vi "TAT_Com_PLC.vi"() -> ()   [LabVIEW 2017]
uses:
  Controls/PLC_Comm_State.ctl
  <vilib>/NI/Modbus Library/API/Master/Modbus Master.lvclass
  <vilib>/NI/Modbus Library/API/Wrapper/Create TCP Master.vi
  Global/PLC_to_Auto.vi
  <vilib>/NI/Modbus Library/API/Wrapper/API Main.lvlib
panel:
  out "PLC IP Address":string
  out "error out 2":errorcluster
  out "error IO":errorcluster
  in  "stop 2":bool
  out "PLC STATUS station 2":bool
  out "error IO 2":errorcluster
  out "Latch Error Case":errorcluster
  out "I/O SCREEN":bool[](array[boolean])
  out "error out":errorcluster
  in  "PLC STATUS station 1":bool
  in  "error in":errorcluster
  in  "stop":bool
  # "STATION 1"
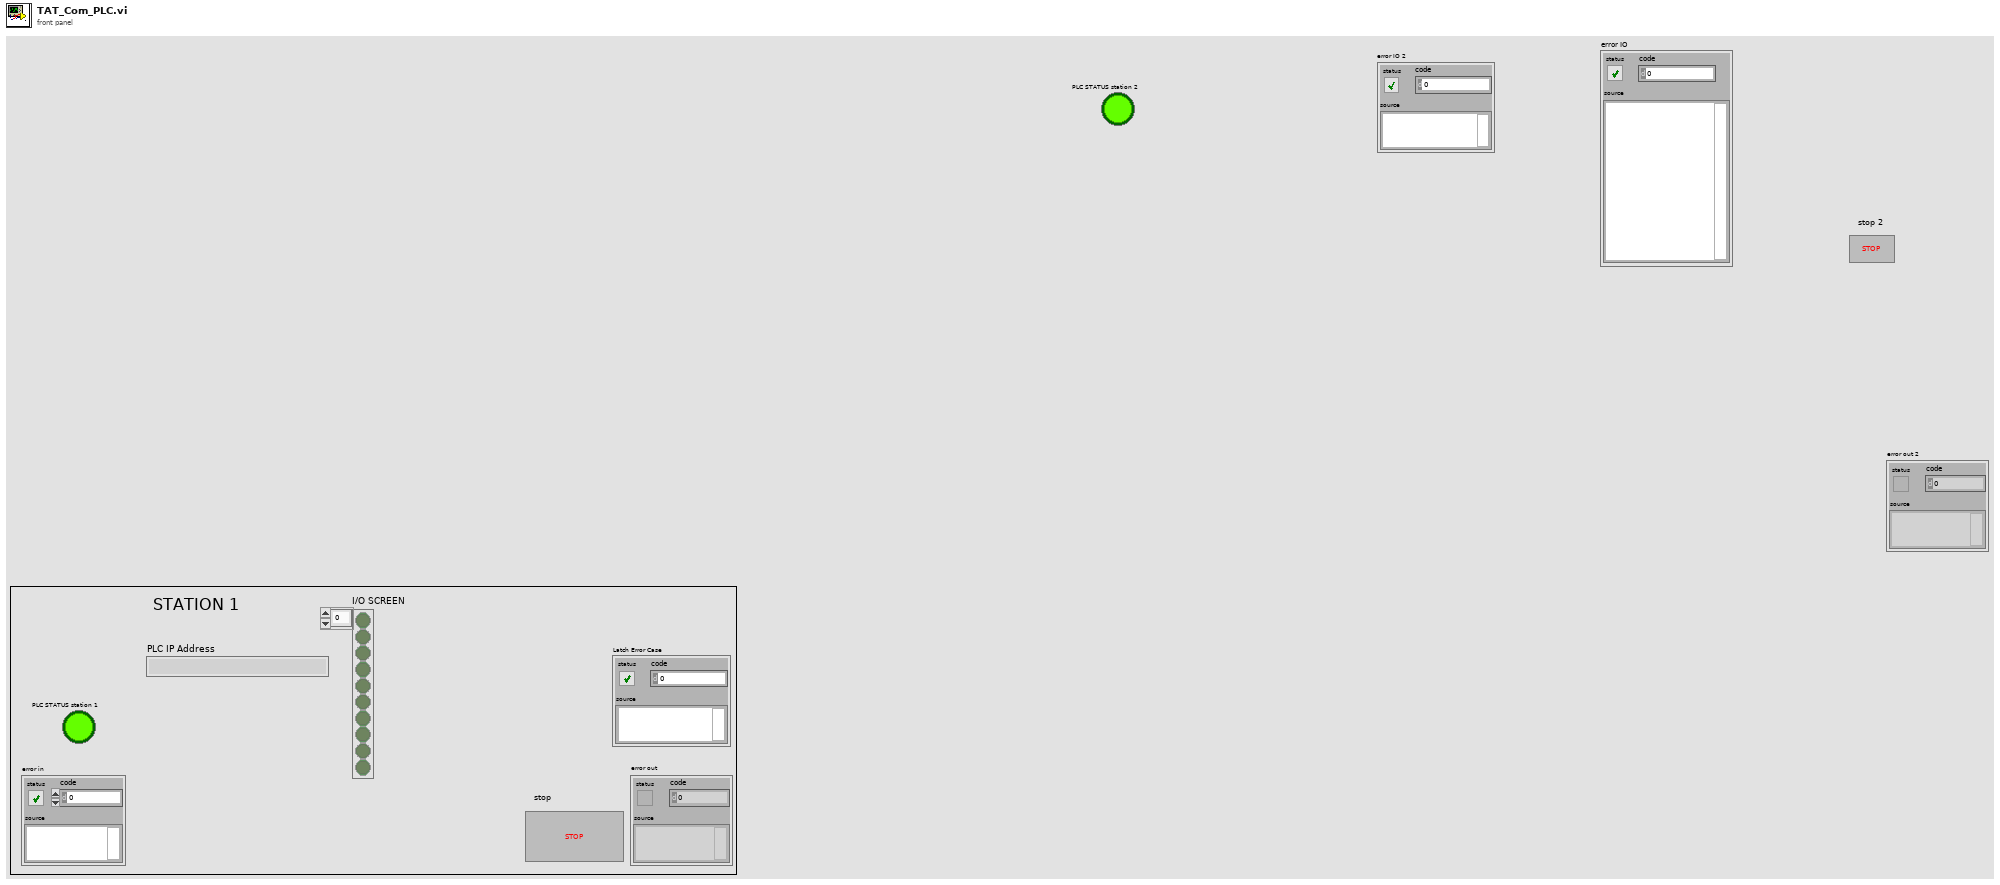
[diagram p1: front panel]
types:
  T1 = typedef "PLC_Comm_State.ctl" = enum16{"Int", "Connect", "Write", "Write2", "Write3", "Read", "Read2", "Read3", "Error", "Disconnect"}
  T2 = enum32{"invalid app kind", "Development System", "Run Time System", "Student Edition", "Embedded LabVIEW", "Evaluation", "Custom"}
  T3 = cluster{"Printer IP":string, "PLC IP Address":string, "Scanner Com":refnum<visa-resource-name>}
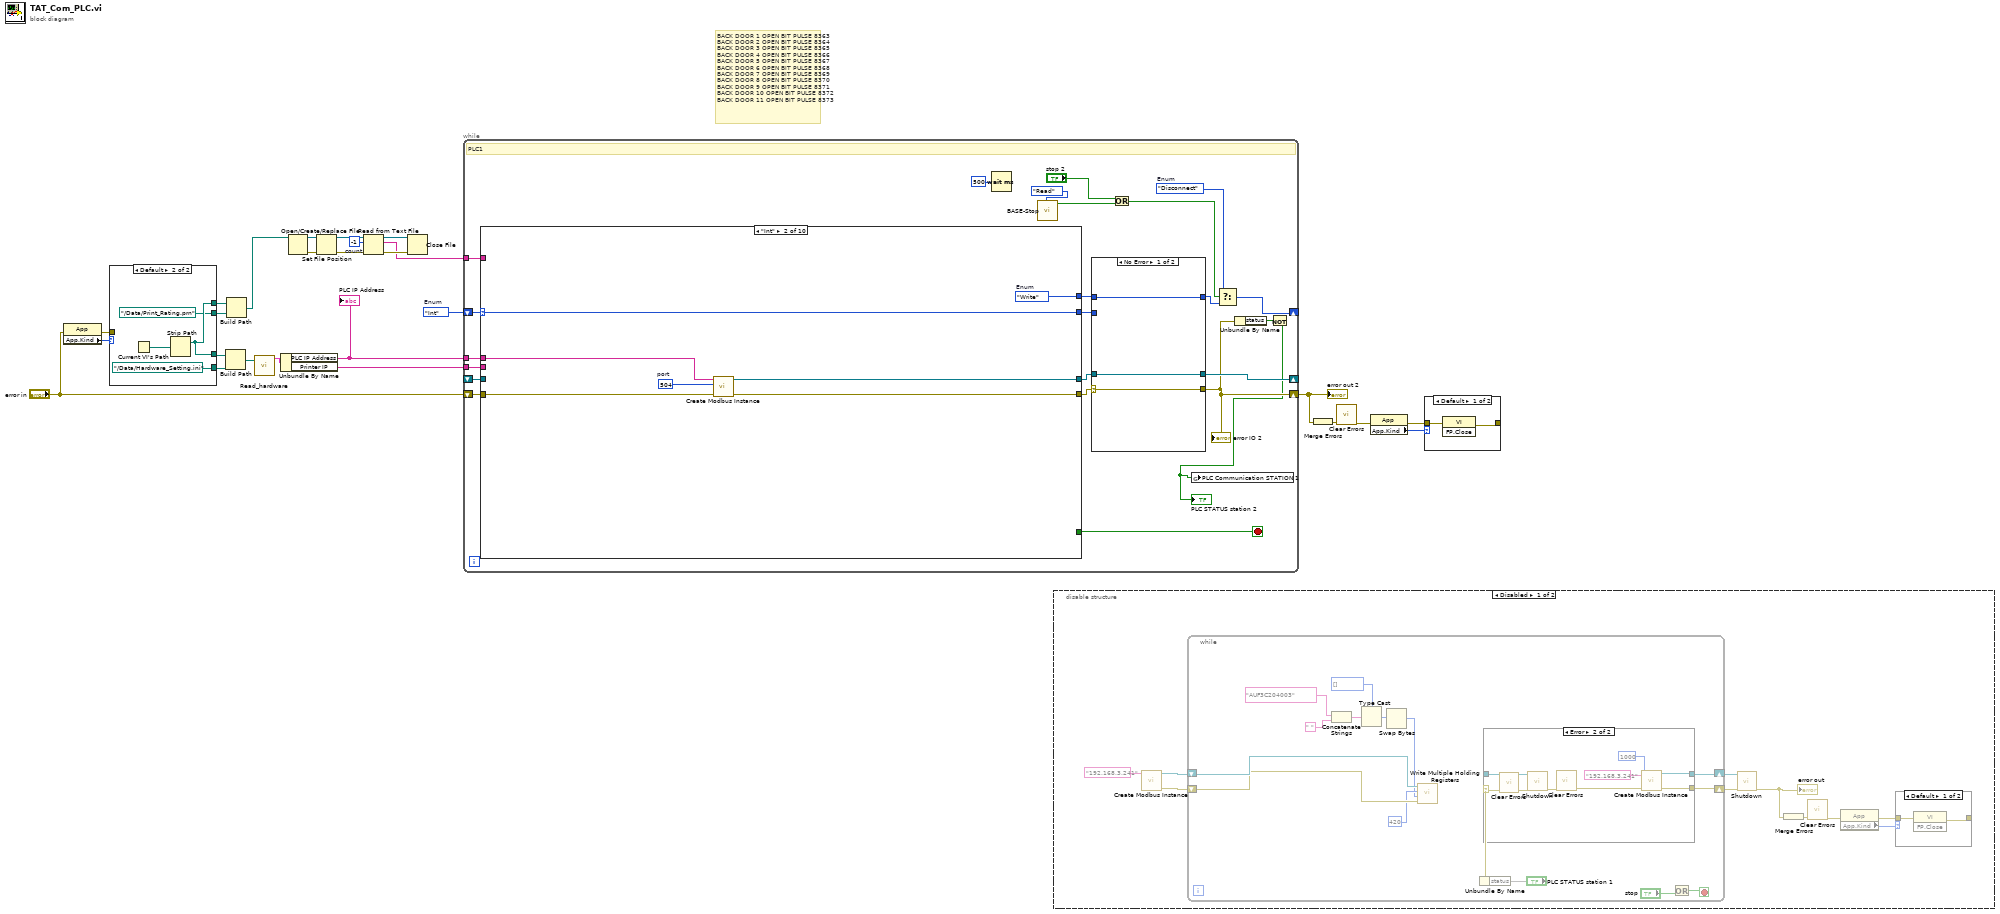
[diagram p0: block diagram]
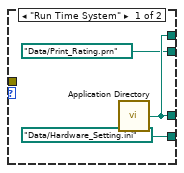
[diagram p2: hidden frame]
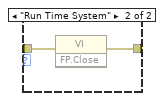
[diagram p4: hidden frame]
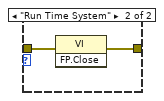
[diagram p6: hidden frame]
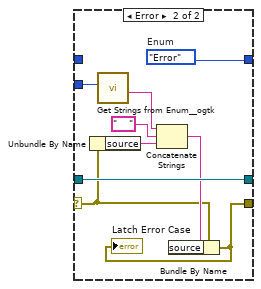
[diagram p7: hidden frame]
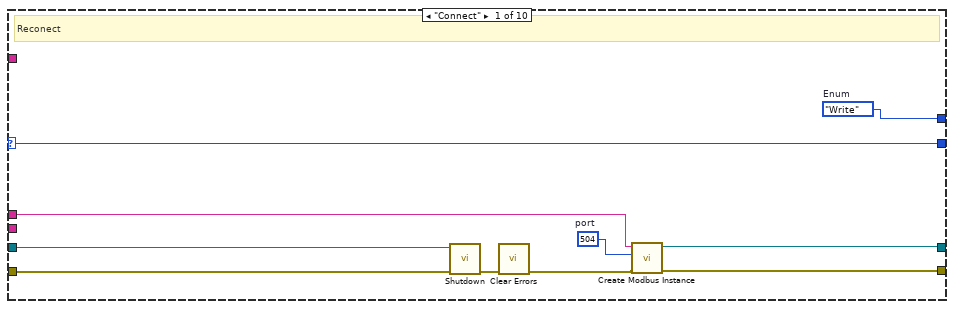
[diagram p8: hidden frame]
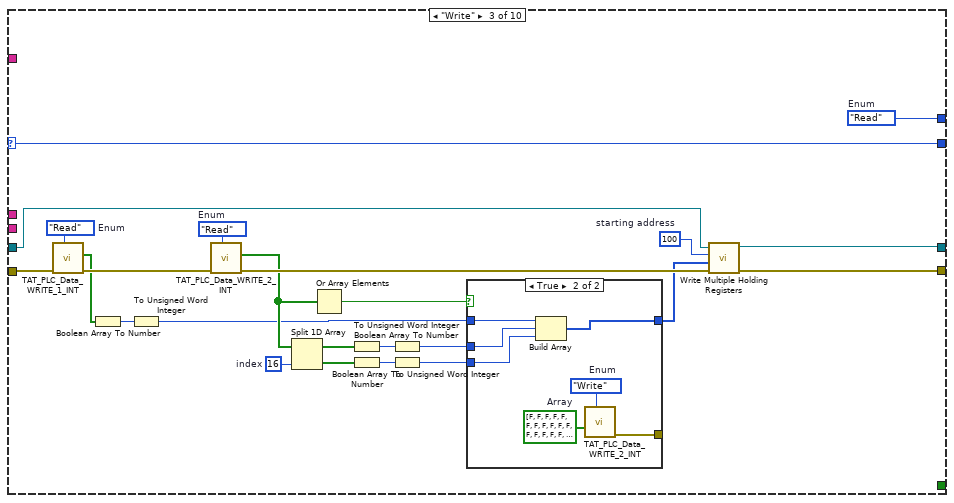
[diagram p9: hidden frame]
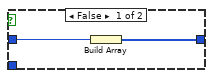
[diagram p10: hidden frame]
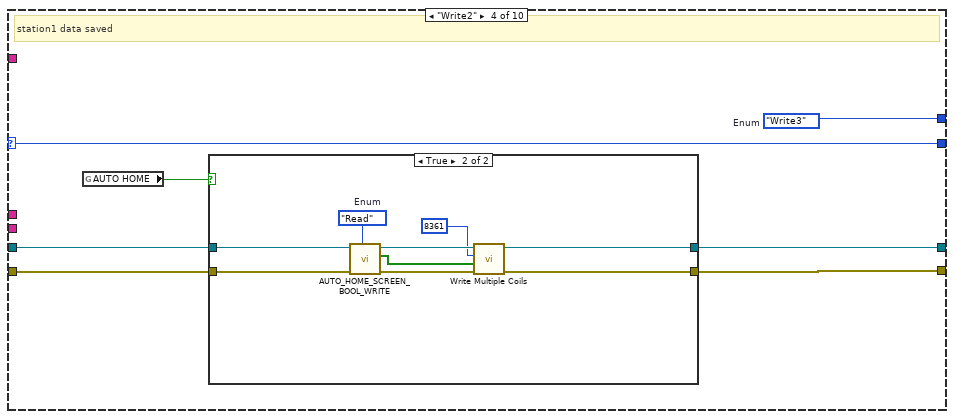
[diagram p11: hidden frame]
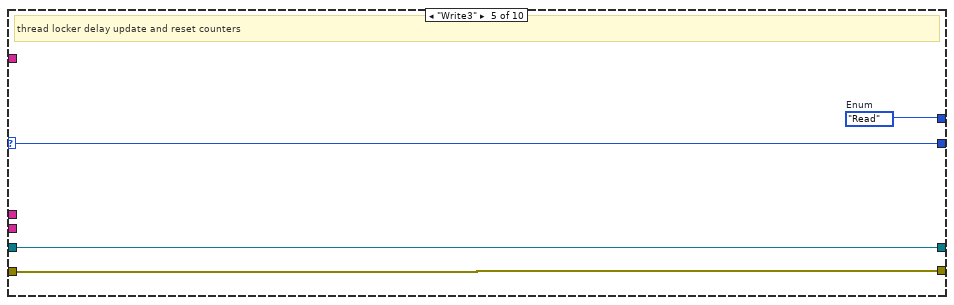
[diagram p13: hidden frame]
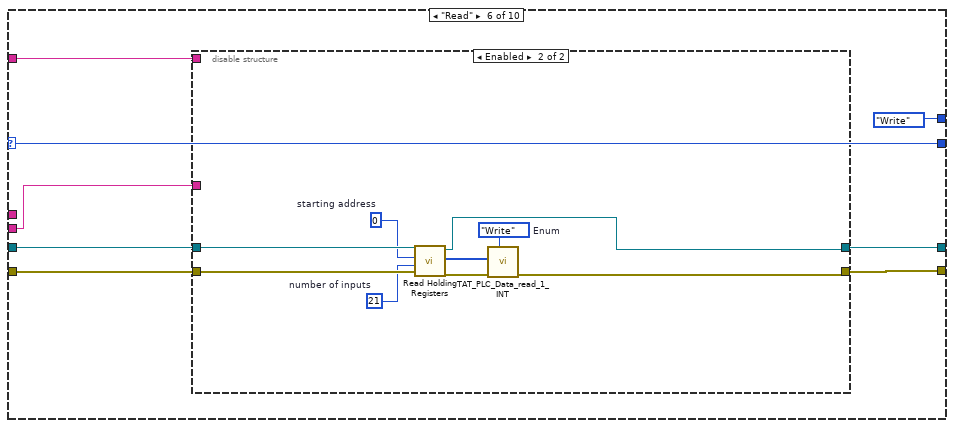
[diagram p14: hidden frame]
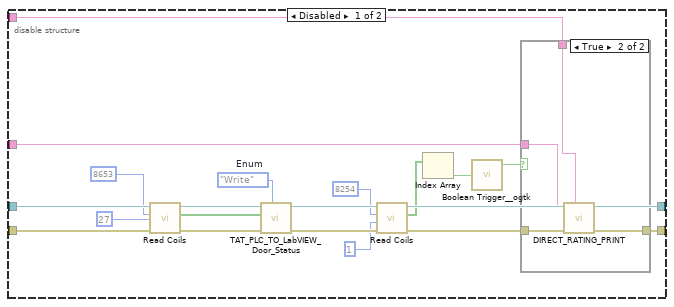
[diagram p15: hidden frame]
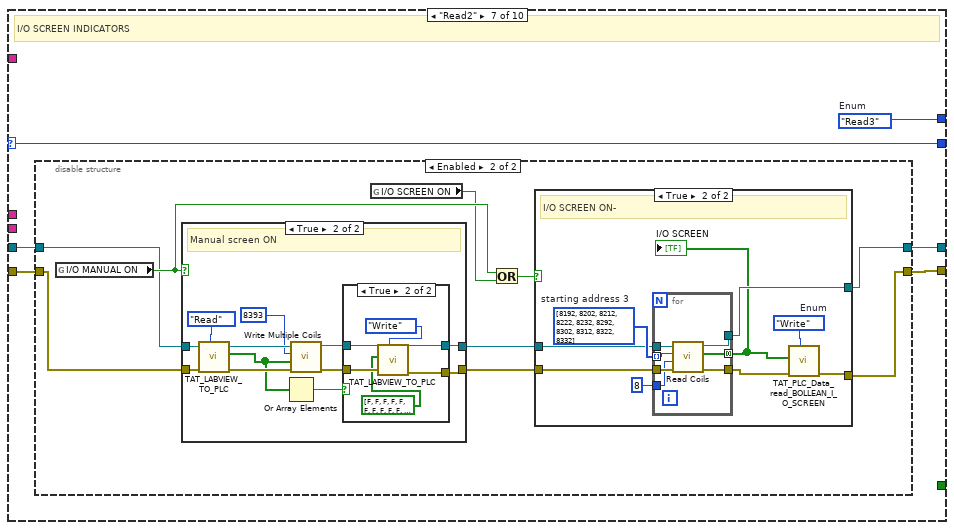
[diagram p17: hidden frame]
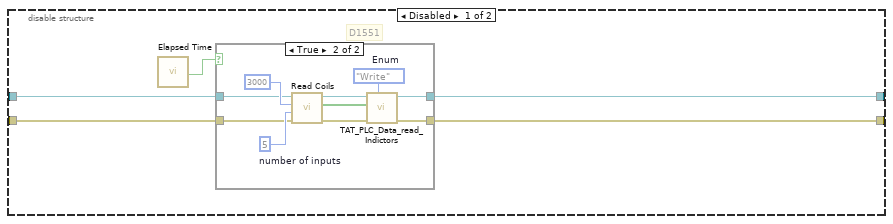
[diagram p18: hidden frame]
diagram:
  w1 = PLC_Comm_State."Int"  # Enum
  w6 = -1  # count
  # "BACK DOOR 1 OPEN BIT\tPULSE\t8363\nBACK DOOR 2 OPEN BIT\tPULSE\t8364\nBACK DOOR 3 OPEN BIT\tPULSE\t8365\nBACK DOOR 4 OPEN BIT\tPULSE\t8366\nBACK DOOR 5 OPEN BIT\tPULSE\t8367\nBACK DOOR 6 OPEN BIT\tPULSE\t8368\nBACK DOOR 7 OPEN BIT\tPULSE\t8369\nBACK DOOR 8 OPEN BIT\tPULSE\t8370\nBACK DOOR 9 OPEN BIT\tPULSE\t8371\nBACK DOOR 10 OPEN BIT\tPULSE\t8372\nBACK DOOR 11 OPEN BIT\tPULSE\t8373"
  n1 = property class="App"(error in="error in") -> (error out=w20:errorcluster, "App.Kind"=w21:T2)  [unwired: 1 in, 1 out]
  n2 = case shown="Default" w21 {
    tunnel: [w28 w31] -> w19
    tunnel: w20 -> [_ _]
    tunnel: [path "Data/Hardware_Setting.ini" ("path") path "../Data/Hardware_Setting.ini" ("path")] -> w18
    tunnel: [w28 w31] -> w5
    tunnel: [path "Data/Print_Rating.prn" ("path") path "../Data/Print_Rating.prn" ("path")] -> w4
    frame "Run Time System" {
      n3 = call <vilib>:"Application Directory.vi"() -> ("Application Directory"=w28:path)
    }
    frame Default {
      n4 = Current VI's Path() -> (path=w33:path)
      n5 = Strip Path(path=w33) -> (stripped path=w31:path)  [unwired: 1 out]
    }
  }
  n6 = Build Path(base path=w19, name or relative path=w18) -> (appended path=w17:path)
  n7 = Build Path(base path=w5, name or relative path=w4) -> (appended path=w3:path)
  n8 = call "Read_hardware.vi"("configuration file path"=w17) -> ("data"=w16:T3)  [unwired: 10 in]
  n9 = Unbundle By Name(w16) -> ("PLC IP Address"=w15:string, "Printer IP"=w13:string)
  "PLC IP Address" <- w15
  n10 = Open/Create/Replace File(file path (use dialog)=w3) -> (refnum out=w11:refnum<file>, error out=w10:errorcluster)  [unwired: 5 in, 1 out]
  n11 = Set File Position(refnum=w11, error in=w10) -> (refnum out=w9:refnum<file>, error out=w12:errorcluster)  [unwired: 2 in]
  n12 = Read from Text File(file (use dialog)=w9, count=w6, error in=w12) -> (refnum out=w8:refnum<file>, text=w2:string, error out=w7:errorcluster)  [unwired: 1 in, 1 out]
  n13 = Close File(refnum=w8, error in=w7) -> ()  [unwired: 2 out]
  n14 = while {
    shift-right: [w47] -> _
    shift-left: w1 -> [w55]
    shift-right: [w42] -> w22
    shift-left: "error in" -> [w54]
    shift-right: [w50] -> _
    shift-left: _ -> [w53]
    tunnel: w15 -> [w52]
    tunnel: w13 -> [w35]
    tunnel: w2 -> [w34]
    stop <- w48 stop-if-true
    w40 = PLC_Comm_State."Disconnect"  # Enum
    # "PLC1"
    n15 = case shown="\"Int\"" w55 {
      selector: w55 -> [w78 w84 w109 w125 w138 w147 w185 w255 w276 w284]
      tunnel: [w75 w80 w94 w122 w136 w143 w181 w253 w277 w281] -> w56
      tunnel: [w73 w81 w96 w119 w137 w141 w182 w251 w278 w279] -> w49
      tunnel: w54 -> [w72 w85 w106 w123 w136 w145 w184 w256 w274 w286]
      tunnel: w53 -> [w70 _ w107 w120 w137 w144 w183 w252 w278 w280]
      tunnel: w52 -> [w74 w82 _ _ _ _ _ _ _ _]
      tunnel: [w77 w83 w108 w124 w139 PLC_Comm_State."Write" ("Enum") w186 w254 w275 w283] -> w51
      tunnel: [_ _ _ _ _ _ _ _ _ TRUE] -> w48
      tunnel: [w78 w84 w109 w125 w138 w147 w185 w255 w276 w284] -> w45
      tunnel: w35 -> [_ _ _ _ _ w142 _ _ _ _]
      tunnel: w34 -> [_ _ _ _ _ w140 _ _ _ _]
      frame "Connect" {
        w69 = u16 504  # port
        w77 = PLC_Comm_State."Write"  # Enum
        # "Reconect"
        n16 = call-dynamic "Shutdown.vi"("error in"=w72, "Modbus master in"=w70) -> ("error out"=w71:errorcluster)  [unwired: 9 in]
        n17 = call <vilib>:"Clear Errors.vi"("error in (no error)"=w71) -> ("error out"=w76:errorcluster)  [unwired: 5 in, 1 out]
        n18 = call-poly <vilib>:"Create Modbus Instance.vi"("error in"=w76, "port (502)"=w69, "address"=w74) -> ("error out"=w75:errorcluster, "TCP master instance"=w73:refnum<class "Modbus Master.lvclass">)  [unwired: 7 in]
      }
      frame "Int" {
        w79 = u16 504  # port
        w83 = PLC_Comm_State."Write"  # Enum
        n19 = call-poly <vilib>:"Create Modbus Instance.vi"("error in"=w85, "port (502)"=w79, "address"=w82) -> ("error out"=w80:errorcluster, "TCP master instance"=w81:refnum<class "Modbus Master.lvclass">)  [unwired: 7 in]
      }
      frame "Write" {
        w89 = u16 100  # starting address
        w101 = 16  # index
        w102 = enum16{"Read", "Write"}."Read"  # Enum
        w104 = enum16{"Read", "Write"}."Read"  # Enum
        w108 = PLC_Comm_State."Read"  # Enum
        n20 = call "TAT_PLC_Data_WRITE_1_INT.vi"("Enum"=w104, "error in (no error)"=w106) -> ("error out"=w105:errorcluster, "Array 2"=w103:bool[])  [unwired: 8 in]
        n21 = Boolean Array To Number(Boolean array=w103) -> (number=w93:u32)
        n22 = To Unsigned Word Integer(number=w93) -> (unsigned 16bit integer=w91:u16)
        n23 = call "TAT_PLC_Data_WRITE_2_INT.vi"("Enum"=w102, "error in (no error)"=w105) -> ("error out"=w95:errorcluster, "Array 2"=w92:bool[])  [unwired: 8 in]
        n24 = Split 1D Array(array=w92, index=w101) -> (first subarray=w98:bool[], second subarray=w97:bool[])
        n25 = Or Array Elements(Boolean array=w92) -> (logical OR=w90:bool)
        n26 = Boolean Array To Number(Boolean array=w98) -> (number=w100:u32)
        n27 = Boolean Array To Number(Boolean array=w97) -> (number=w99:u32)
        n28 = To Unsigned Word Integer(number=w100) -> (unsigned 16bit integer=w87:u16)
        n29 = To Unsigned Word Integer(number=w99) -> (unsigned 16bit integer=w86:u16)
        n30 = case shown="True" w90 {
          tunnel: w91 -> [w111 w118]
          tunnel: [w110 w117] -> w88
          tunnel: w87 -> [_ w116]
          tunnel: w86 -> [_ w115]
          tunnel: [_ w113] -> _
          frame False {
            n31 = Build Array(w111) -> (w110:u16[])
          }
          frame True {
            w112 = bool[] [FALSE, FALSE, FALSE, FALSE, FALSE, FALSE, FALSE, FALSE, FALSE, FALSE, FALSE, FALSE, FALSE, FALSE, FALSE, FALSE, FALSE, FALSE, FALSE, FALSE, FALSE, FALSE, FALSE, FALSE, FALSE, FALSE, FALSE, FALSE, FALSE, FALSE, FALSE, FALSE]  # Array
            w114 = enum16{"Read", "Write"}."Write"  # Enum
            n32 = Build Array(w118, w116, w115) -> (w117:u16[])
            n33 = call "TAT_PLC_Data_WRITE_2_INT.vi"("Enum"=w114, "Array"=w112) -> ("error out"=w113:errorcluster)  [unwired: 8 in, 1 out]
          }
        }
        n34 = call-dynamic "Write Multiple Holding Registers.vi"("error in"=w95, "registers to write"=w88, "starting address"=w89, "Modbus master in"=w107) -> ("error out"=w94:errorcluster, "Modbus master out"=w96:refnum<class "Modbus Master.lvclass">)  [unwired: 6 in]
      }
      frame "Write2" {
        w124 = PLC_Comm_State."Write3"  # Enum
        # "station1 data saved"
        n35 = global read "PLC_to_Auto.vi" "AUTO HOME"() -> (w121:bool)
        n36 = case shown="True" w121 {
          tunnel: w123 -> [w127 w130]
          tunnel: [w127 w135] -> w122
          tunnel: w120 -> [w126 w134]
          tunnel: [w126 w133] -> w119
          frame False {
          }
          frame True {
            w131 = enum16{"Read", "Write"}."Read"  # Enum
            n37 = call "AUTO_HOME_SCREEN_BOOL_WRITE.vi"("Enum"=w131, "error in (no error)"=w130) -> ("error out"=w129:errorcluster, "Array 2"=w128:bool[])  [unwired: 8 in]
            n38 = call-dynamic "Write Multiple Coils.vi"("error in"=w129, "coils to write"=w128, "starting address"=u16 8361, "Modbus master in"=w134) -> ("error out"=w135:errorcluster, "Modbus master out"=w133:refnum<class "Modbus Master.lvclass">)  [unwired: 6 in]
          }
        }
      }
      frame "Write3" {
        w139 = PLC_Comm_State."Read"  # Enum
        # "thread locker delay update and reset counters"
      }
      frame "Read" {
        n39 = disable-structure shown="Enabled" {
          disable-tunnel: w145 -> [w164 w180]
          disable-tunnel: w144 -> [w163 w179]
          disable-tunnel: [w159 w174] -> w143
          disable-tunnel: w142 -> [w157 _]
          disable-tunnel: [w155 w175] -> w141
          disable-tunnel: w140 -> [w148 _]
          frame Disabled {
            w166 = enum16{"Read", "Write"}."Write"  # Enum
            n40 = call-dynamic "Read Coils.vi"("error in"=w164, "number of inputs"=u16 27, "starting address"=u16 8653, "Modbus master in"=w163) -> ("error out"=w165:errorcluster, "coils"=w160:bool[], "Modbus master out"=w156:refnum<class "Modbus Master.lvclass">)  [unwired: 5 in]
            n41 = call "TAT_PLC_TO_LabVIEW_Door_Status.vi"("Enum"=w166, "error in (no error)"=w165, "Array"=w160) -> ("error out"=w154:errorcluster)  [unwired: 7 in, 1 out]
            n42 = call-dynamic "Read Coils.vi"("error in"=w154, "number of inputs"=u16 1, "starting address"=u16 8254, "Modbus master in"=w156) -> ("error out"=w153:errorcluster, "coils"=w150:bool[], "Modbus master out"=w155:refnum<class "Modbus Master.lvclass">)  [unwired: 5 in]
            n43 = Index Array(array=w150) -> (element=w149:bool)  [unwired: 1 in]
            n44 = call <userlib>:"Boolean Trigger__ogtk.vi"("Boolean Input"=w149) -> ("Rising Edge"=w158:bool)  [unwired: 1 in, 1 out]
            n45 = case shown="True" w158 {
              tunnel: w153 -> [w167 w171]
              tunnel: [w167 w170] -> w159
              tunnel: w157 -> [_ w169]
              tunnel: w148 -> [_ w168]
              frame False {
              }
              frame True {
                n46 = call "DIRECT_RATING_PRINT.vi"("PRN Data"=w168, "error in"=w171, "Printer IP"=w169) -> ("error out"=w170:errorcluster)  [unwired: 8 in]
              }
            }
          }
          frame Enabled {
            w172 = u16 21  # number of inputs
            w173 = u16 0  # starting address
            w178 = enum16{"Read", "Write"}."Write"  # Enum
            n47 = call-dynamic "Read Holding Registers.vi"("error in"=w180, "number of inputs"=w172, "starting address"=w173, "Modbus master in"=w179) -> ("error out"=w177:errorcluster, "register values"=w176:u16[], "Modbus master out"=w175:refnum<class "Modbus Master.lvclass">)  [unwired: 5 in]
            n48 = call "TAT_PLC_Data_read_1_INT.vi"("Enum"=w178, "error in (no error)"=w177, "Array"=w176) -> ("error out"=w174:errorcluster)  [unwired: 7 in, 1 out]
          }
        }
      }
      frame "Read2" {
        w186 = PLC_Comm_State."Read3"  # Enum
        # "I/O SCREEN INDICATORS"
        n49 = disable-structure shown="Enabled" {
          disable-tunnel: w184 -> [w191 w206]
          disable-tunnel: w183 -> [w190 w203]
          disable-tunnel: [w189 w204] -> w182
          disable-tunnel: [w188 w205] -> w181
          frame Disabled {
            # "D1551"
            n50 = call "Elapsed Time"() -> ("Time has Elapsed"=w187:bool)  [unwired: 12 in, 7 out]
            n51 = case shown="True" w187 {
              tunnel: w191 -> [w192 w200]
              tunnel: w190 -> [w193 w199]
              tunnel: [w193 w198] -> w189
              tunnel: [w192 w194] -> w188
              frame False {
              }
              frame True {
                w197 = enum16{"Read", "Write"}."Write"  # Enum
                w202 = u16 5  # number of inputs
                n52 = call-dynamic "Read Coils.vi"("error in"=w200, "number of inputs"=w202, "starting address"=u16 3000, "Modbus master in"=w199) -> ("error out"=w195:errorcluster, "coils"=w196:bool[], "Modbus master out"=w198:refnum<class "Modbus Master.lvclass">)  [unwired: 5 in]
                n53 = call "TAT_PLC_Data_read_Indictors.vi"("Enum"=w197, "error in (no error)"=w195, "Array"=w196) -> ("error out"=w194:errorcluster)  [unwired: 7 in, 1 out]
              }
            }
          }
          frame Enabled {
            n54 = global read "PLC_to_Auto.vi" "I/O MANUAL ON"() -> (w211:bool)
            n55 = case shown="True" w211 {
              tunnel: w206 -> [w212 w221]
              tunnel: [w212 w216] -> w207
              tunnel: [w213 w215] -> w208
              tunnel: w203 -> [w213 w224]
              frame False {
                # "Manual screen OFF"
              }
              frame True {
                # "Manual screen ON"
                n56 = call "TAT_LABVIEW_TO_PLC.vi"("Enum"=enum16{"Read", "Write"}."Read", "error in (no error)"=w221) -> ("error out"=w220:errorcluster, "Array 2"=w219:bool[])  [unwired: 8 in]
                n57 = Or Array Elements(Boolean array=w219) -> (logical OR=w218:bool)
                n58 = call-dynamic "Write Multiple Coils.vi"("error in"=w220, "coils to write"=w219, "starting address"=u16 8393, "Modbus master in"=w224) -> ("error out"=w217:errorcluster, "Modbus master out"=w214:refnum<class "Modbus Master.lvclass">)  [unwired: 6 in]
                n59 = case shown="True" w218 {
                  tunnel: w217 -> [w225 w231]
                  tunnel: [w225 w230] -> w216
                  tunnel: [w226 w229] -> w215
                  tunnel: w214 -> [w226 w229]
                  frame False {
                  }
                  frame True {
                    n60 = call "TAT_LABVIEW_TO_PLC.vi"("Enum"=enum16{"Read", "Write"}."Write", "error in (no error)"=w231, "Array"=bool[] [FALSE, FALSE, FALSE, FALSE, FALSE, FALSE, FALSE, FALSE, FALSE, FALSE, FALSE, FALSE, FALSE, FALSE, FALSE, FALSE, FALSE, FALSE, FALSE, FALSE, FALSE, FALSE, FALSE, FALSE, FALSE, FALSE, FALSE, FALSE, FALSE, FALSE, FALSE, FALSE, FALSE, FALSE, FALSE, FALSE, FALSE, FALSE, FALSE, FALSE, FALSE, FALSE, FALSE, FALSE, FALSE]) -> ("error out"=w230:errorcluster)  [unwired: 7 in, 1 out]
                  }
                }
              }
            }
            n61 = global read "PLC_to_Auto.vi" "I/O SCREEN ON"() -> (w209:bool)
            n62 = Or(x=w211, y=w209) -> (x .or. y?=w210:bool)
            n63 = case shown="True" w210 {
              tunnel: [w232 w237] -> w205
              tunnel: [w233 w242] -> w204
              tunnel: w207 -> [w232 w240]
              tunnel: w208 -> [w233 w239]
              frame False {
                # "I/O SCREEN Off-"
              }
              frame True {
                w241 = u16[] [8192, 8202, 8212, 8222, 8232, 8292, 8302, 8312, 8322, 8332]  # starting address 3
                w238 = enum16{"Read", "Write"}."Write"  # Enum
                # "I/O SCREEN ON-"
                n64 = for {
                  tunnel: u16 8 ("number of inputs") -> [w246]
                  tunnel: w241 -> [w245] mode=indexing
                  tunnel: w240 -> [w249]
                  tunnel: [w244] -> w236
                  tunnel: w239 -> [w248]
                  tunnel: [w247] -> w242
                  tunnel: [w243] -> w235 mode=concatenating
                  n65 = call-dynamic "Read Coils.vi"("error in"=w249, "number of inputs"=w246, "starting address"=w245, "Modbus master in"=w248) -> ("error out"=w244:errorcluster, "coils"=w243:bool[], "Modbus master out"=w247:refnum<class "Modbus Master.lvclass">)  [unwired: 5 in]
                }
                "I/O SCREEN" <- w235
                n66 = call "TAT_PLC_Data_read_BOLLEAN_I_O_SCREEN.vi"("Enum"=w238, "error in (no error)"=w236, "Array"=w235) -> ("error out"=w237:errorcluster)  [unwired: 7 in, 1 out]
              }
            }
          }
        }
      }
      frame "Read3" {
        w254 = PLC_Comm_State."Write"  # Enum
        # "AUTO HOME SCREEN"
        n67 = global read "PLC_to_Auto.vi" "AUTO HOME"() -> (w250:bool)
        n68 = case shown="True" w250 {
          tunnel: w256 -> [w257 w273]
          tunnel: [w257 w264] -> w253
          tunnel: w252 -> [w258 w272]
          tunnel: [w258 w262] -> w251
          frame False {
          }
          frame True {
            w266 = enum16{"Read", "Write"}."Write"  # Enum
            w268 = enum16{"Read", "Write"}."Write"  # Enum
            n69 = call-dynamic "Read Holding Registers.vi"("error in"=w273, "number of inputs"=u16 58, "starting address"=u16 201, "Modbus master in"=w272) -> ("error out"=w269:errorcluster, "register values"=w267:u16[], "Modbus master out"=w263:refnum<class "Modbus Master.lvclass">)  [unwired: 5 in]
            n70 = call "AUTO_HOME_SCREEN.vi"("Enum"=w268, "error in (no error)"=w269, "Array"=w267) -> ("error out"=w265:errorcluster)  [unwired: 7 in, 1 out]
            n71 = call-dynamic "Read Coils.vi"("error in"=w265, "number of inputs"=u16 7, "starting address"=u16 8255, "Modbus master in"=w263) -> ("error out"=w264:errorcluster, "coils"=w259:bool[], "Modbus master out"=w262:refnum<class "Modbus Master.lvclass">)  [unwired: 5 in]
            n72 = call "AUTO_HOME_SCREEN_BOOL.vi"("Enum"=w266, "Array"=w259) -> ()  [unwired: 8 in, 2 out]
          }
        }
      }
      frame "Error" {
        w275 = PLC_Comm_State."Connect"  # Enum
        n73 = call <vilib>:"Clear Errors.vi"("error in (no error)"=w274) -> ("error out"=w277:errorcluster)  [unwired: 5 in, 1 out]
        "error IO" <- w274
      }
      frame "Disconnect" {
        w279 = refnum<class "Modbus Master.lvclass"> refnum  # Modbus master out
        w283 = PLC_Comm_State."Disconnect"  # Enum
        n74 = call <vilib>:"Clear Errors.vi"("error in (no error)"=w286) -> ("error out"=w282:errorcluster)  [unwired: 5 in, 1 out]
        n75 = call-dynamic "Shutdown.vi"("error in"=w282, "Modbus master in"=w280) -> ("error out"=w281:errorcluster)  [unwired: 9 in]
      }
    }
    n76 = Wait (ms)(milliseconds to wait=u32 500) -> ()  [unwired: 1 out]
    n77 = call "BASE-Stop.vi"("Enum"=enum16{"Read", "Write"}."Read") -> ("Stop"=w38:bool)  [unwired: 10 in]
    n78 = case shown="No Error" w56 {
      selector: w56 -> [w59 w62]
      tunnel: [w59 w60] -> w42
      tunnel: [w58 w61] -> w46
      tunnel: w51 -> [w58 _]
      tunnel: [w57 w68] -> w50
      tunnel: w49 -> [w57 w68]
      tunnel: w45 -> [_ w66]
      frame No Error {
      }
      frame Error {
        w61 = PLC_Comm_State."Error"  # Enum
        n79 = Unbundle By Name(w62) -> ("source"=w67:string)
        n80 = call <userlib>:"Get Strings from Enum__ogtk.vi"("Enum"=w66) -> ("String Value"=w65:string)  [unwired: 7 in, 3 out]
        n81 = Concatenate Strings(w65, "    " ("string"), w67) -> (w63:string)
        n82 = Bundle By Name(cluster=w62, "source"=w63) -> (w60:errorcluster)
        "Latch Error Case" <- w60
      }
    }
    "error IO 2" <- w42
    n83 = Or(x="stop 2", y=w38) -> (x .or. y?=w44:bool)
    n84 = Select(t=w40, s=w44, f=w46) -> (s? t:f=w47:T1)
    n85 = Unbundle By Name(w42) -> ("status"=w43:bool)
    n86 = Not(x=w43) -> (.not. x?=w37:bool)
    "PLC STATUS station 2" <- w37
    n87 = global write "PLC_to_Auto.vi" "PLC Communication STATION 1"(w37) -> ()
  }
  "error out 2" <- w22
  n88 = disable-structure shown="Disabled" {
    frame Disabled {
      n89 = call-poly <vilib>:"Create Modbus Instance.vi"("address"="192.168.3.241") -> ("error out"=w291:errorcluster, "TCP master instance"=w290:refnum<class "Modbus Master.lvclass">)  [unwired: 9 in]
      n90 = while {
        shift-right: [w312] -> w295
        shift-left: w290 -> [w306]
        shift-right: [w311] -> w294
        shift-left: w291 -> [w304]
        stop <- w313 stop-if-true
        n91 = Concatenate Strings("AUF3C204003", " ") -> (w297:string)
        n92 = Type Cast(type=u16[] [] ("Register"), x=w297) -> (*(type *) &x=w300:u16[])
        n93 = Swap Bytes(anything=w300) -> (byte swapped=w299:u16[])
        n94 = call-dynamic "Write Multiple Holding Registers.vi"("error in"=w304, "registers to write"=w299, "starting address"=u16 420, "Modbus master in"=w306) -> ("error out"=w303:errorcluster, "Modbus master out"=w305:refnum<class "Modbus Master.lvclass">)  [unwired: 6 in]
        n95 = case shown="Error" w308 {
          selector: [w315 w325] -> w308
          tunnel: [w316 w323] -> w310
          tunnel: [w316 w319] -> w312
          tunnel: [w315 w318] -> w311
          frame No Error {
          }
          frame Error {
            n96 = call <vilib>:"Clear Errors.vi"("error in (no error)"=w325) -> ("error out"=w324:errorcluster)  [unwired: 5 in, 1 out]
            n97 = call-dynamic "Shutdown.vi"("error in"=w324, "Modbus master in"=w323) -> ("error out"=w322:errorcluster)  [unwired: 9 in]
            n98 = call <vilib>:"Clear Errors.vi"("error in (no error)"=w322) -> ("error out"=w320:errorcluster)  [unwired: 5 in, 1 out]
            n99 = call-poly <vilib>:"Create Modbus Instance.vi"("error in"=w320, "connect timeout ms"=1000, "address"="192.168.3.241") -> ("error out"=w318:errorcluster, "TCP master instance"=w319:refnum<class "Modbus Master.lvclass">)  [unwired: 7 in]
          }
        }
        n100 = Unbundle By Name(w308) -> ("status"=→"PLC STATUS station 1")
        n101 = Or(y="stop") -> (x .or. y?=w313:bool)  [unwired: 1 in]
      }
      n102 = call-dynamic "Shutdown.vi"("error in"=w294, "Modbus master in"=w295) -> ("error out"=w288:errorcluster)  [unwired: 9 in]
      "error out" <- w288
      n103 = Merge Errors(w288) -> (w287:errorcluster)
      n104 = call <vilib>:"Clear Errors.vi"("error in (no error)"=w287) -> ("error out"=w289:errorcluster)  [unwired: 5 in, 1 out]
      n105 = property class="App"(error in=w289) -> (error out=w292:errorcluster, "App.Kind"=w293:T2)  [unwired: 1 in, 1 out]
      n106 = case shown="Default" w293 {
        tunnel: w292 -> [w327 w329]
        tunnel: [w326 w328] -> _
        frame Default {
          n107 = invoke class="VI" method="FP.Close"(error in=w327) -> (error out=w326:errorcluster)  [unwired: 2 in, 2 out]
        }
        frame "Run Time System" {
          n108 = invoke class="VI" method="FP.Close"(error in=w329) -> (error out=w328:errorcluster)  [unwired: 2 in, 2 out]
        }
      }
    }
    frame Enabled {
    }
  }
  n109 = Merge Errors(w22) -> (w26:errorcluster)
  n110 = call <vilib>:"Clear Errors.vi"("error in (no error)"=w26) -> ("error out"=w25:errorcluster)  [unwired: 5 in, 1 out]
  n111 = property class="App"(error in=w25) -> (error out=w24:errorcluster, "App.Kind"=w23:T2)  [unwired: 1 in, 1 out]
  n112 = case shown="Default" w23 {
    tunnel: w24 -> [w331 w333]
    tunnel: [w330 w332] -> _
    frame Default {
      n113 = invoke class="VI" method="FP.Close"(error in=w331) -> (error out=w330:errorcluster)  [unwired: 2 in, 2 out]
    }
    frame "Run Time System" {
      n114 = invoke class="VI" method="FP.Close"(error in=w333) -> (error out=w332:errorcluster)  [unwired: 2 in, 2 out]
    }
  }
